vi "TCP Generic Ack.vi"(8 "error in (no error)":errorcluster, 11 "connection ID":refnum<k5>) -> (0 "error out":errorcluster, 3 "connection ID out":refnum<k5>)   [LabVIEW 2020]
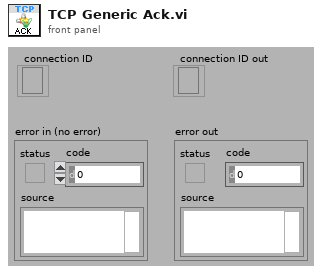
[diagram p1: front panel]
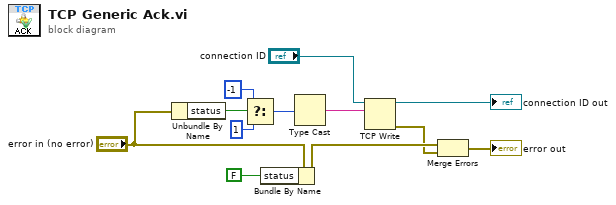
[diagram p0: block diagram]
diagram:
  n1 = Unbundle By Name("error in (no error)") -> ("status"=w10:bool)
  n2 = Select(t=-1, s=w10, f=1) -> (s? t:f=w7:i32)
  n3 = Bundle By Name(cluster="error in (no error)", "status"=FALSE) -> (w4:errorcluster)
  n4 = Type Cast(x=w7) -> (*(type *) &x=w12:string)  [unwired: 1 in]
  n5 = TCP Write(connection ID="connection ID", data in=w12) -> (connection ID out=→"connection ID out":refnum<k5>, error out=w1:errorcluster)  [unwired: 2 in, 1 out]
  n6 = Merge Errors(w4, w1) -> (→"error out":errorcluster)
